vi "Post-Build Action.vi"(5 "Files Generated by Build":path[](array[path]), 6 "Top Level/Always Included VIs":path[](array[path]), 7 "Destination Path":path, 8 "error in (no error)":errorcluster, 9 "Target Name":string, 10 "Build Specification Name":string, 11 "Project Path":path) -> (0 "error out":errorcluster)   [LabVIEW 2023]
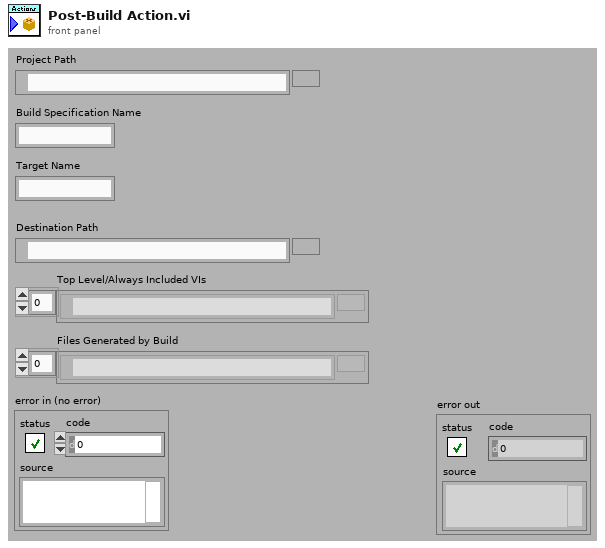
[diagram p1: front panel]
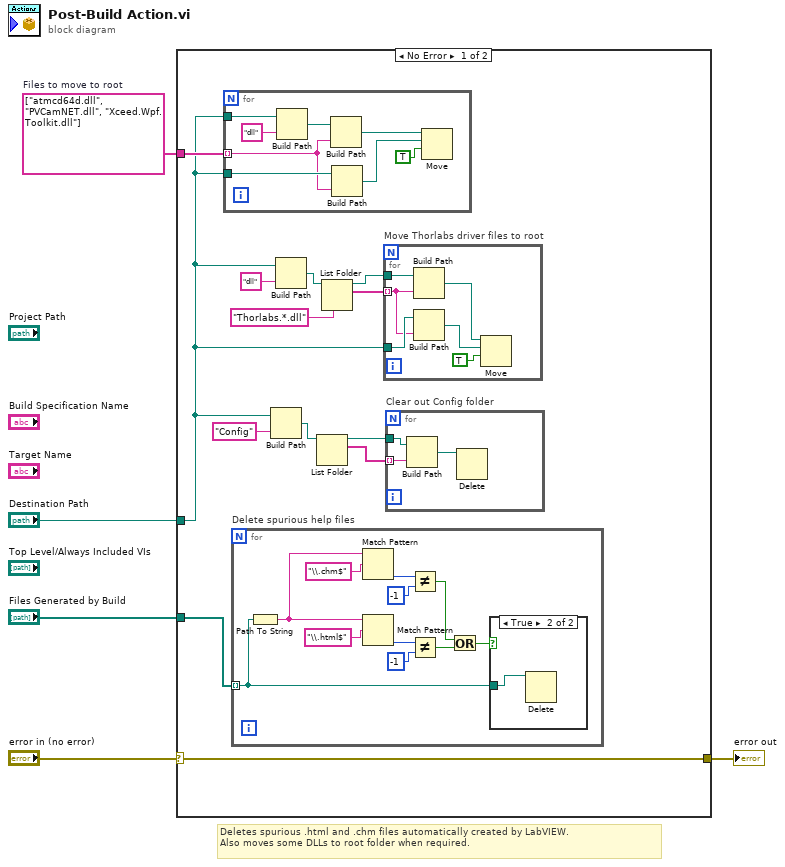
[diagram p0: block diagram]
diagram:
  w1 = string[] ["atmcd64d.dll", "PVCamNET.dll", "Xceed.Wpf.Toolkit.dll"]  # Files to move to root
  # "Deletes spurious .html and .chm files automatically created by LabVIEW.\nAlso moves some DLLs to root folder when required."
  n1 = case shown="No Error" "error in (no error)" {
    selector: "error in (no error)" -> [w18 w48]
    tunnel: [w18 w48] -> w4
    tunnel: "Destination Path" -> [w9 _]
    tunnel: "Files Generated by Build" -> [w17 _]
    tunnel: w1 -> [w11 _]
    frame No Error {
      n2 = for {
        tunnel: w9 -> [w28]
        tunnel: w11 -> [w24] mode=indexing
        tunnel: w9 -> [w25]
        n3 = Build Path(base path=w28, name or relative path="dll" ("format string")) -> (appended path=w27:path)
        n4 = Build Path(base path=w27, name or relative path=w24) -> (appended path=w26:path)
        n5 = Build Path(base path=w25, name or relative path=w24) -> (appended path=w23:path)
        n6 = Move(source path=w26, 9:TRUE ("overwrite (F)"), 10:w23) -> ()  [unwired: 2 in, 3 out]
      }
      n7 = for "Delete spurious help files" {
        tunnel: w17 -> [w37] mode=indexing
        n8 = Path To String(path=w37) -> (string=w36:string)
        n9 = Match Pattern(string=w36, regular expression="\\.chm$") -> (offset past match=w45:i32)  [unwired: 1 in, 3 out]
        n10 = Match Pattern(string=w36, regular expression="\\.html$") -> (offset past match=w42:i32)  [unwired: 1 in, 3 out]
        n11 = Not Equal?(x=w45, y=-1) -> (x != y?=w40:bool)
        n12 = Not Equal?(x=w42, y=-1) -> (x != y?=w39:bool)
        n13 = Or(x=w40, y=w39) -> (x .or. y?=w38:bool)
        n14 = case shown="True" w38 {
          tunnel: w37 -> [_ w47]
          frame False {
          }
          frame True {
            n15 = Delete(path (use dialog)=w47) -> ()  [unwired: 4 in, 3 out]
          }
        }
      }
      n16 = Build Path(base path=w9, name or relative path="Config" ("format string")) -> (appended path=w8:path)
      n17 = Build Path(base path=w9, name or relative path="dll" ("format string")) -> (appended path=w15:path)
      n18 = List Folder(path=w8) -> (path out=w7:path, filenames=w6:string[])  [unwired: 3 in, 2 out]
      n19 = List Folder(path=w15, pattern="Thorlabs.*.dll" ("format string")) -> (path out=w12:path, filenames=w13:string[])  [unwired: 2 in, 2 out]
      n20 = for "Move Thorlabs driver files to root" {
        tunnel: w13 -> [w31] mode=indexing
        tunnel: w12 -> [w35]
        tunnel: w9 -> [w32]
        n21 = Build Path(base path=w35, name or relative path=w31) -> (appended path=w34:path)
        n22 = Build Path(base path=w32, name or relative path=w31) -> (appended path=w30:path)
        n23 = Move(source path=w34, 9:TRUE ("overwrite"), 10:w30) -> ()  [unwired: 2 in, 3 out]
      }
      n24 = for "Clear out Config folder" {
        tunnel: w7 -> [w20]
        tunnel: w6 -> [w21] mode=indexing
        n25 = Build Path(base path=w20, name or relative path=w21) -> (appended path=w19:path)
        n26 = Delete(path (use dialog)=w19) -> ()  [unwired: 4 in, 3 out]
      }
    }
    frame Error {
    }
  }
  "error out" <- w4
